vi "自动.vi"() -> ()   [LabVIEW 2017]
uses:
  <vilib>/Platform/TimedLoop/XDataNode/XDataNode.xnode
  <vilib>/Platform/TimedLoop/XDataNode/nitl_modes.ctl
  <vilib>/Platform/TimedLoop/XDataNode/XDNodeRunTimeDep.lvlib
  <vilib>/Platform/TimedLoop/XDataNode/wakeup.ctl
  <vilib>/Platform/TimedLoop/XDataNode/timing_clust.ctl
  <vilib>/rvi/interface/nirviCloseFPGA/nirviCloseFPGA.xnode
  <vilib>/myRIO/Instrument Drivers/Utilities/Utilities.lvlib
  <vilib>/FPGAPlugInAG/Dynamic/niLvFpga_Close_Dynamic.vi
panel:
  in  "开始":bool
  in  "枚举":enum16{"等待", "前进", "减速", "停止"}(ring)
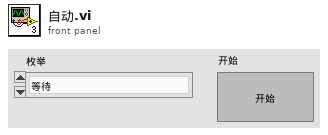
[diagram p1: front panel]
types:
  T1 = typedef "PWM.lvlib/PWM Reference.ctl" = cluster{"myRIO Reference":T2, "PWM Channels Enum":T6, "PWM Configuration":T7}
  T2 = typedef "myRIO Generic Hardware Reference.ctl" = cluster{"myRIO Model":T3, "myRIO Hardware Reference":T4}
  T3 = typedef "Hardware Version Enum.ctl" = enum16{"Unknown", "myRIO-1900", "myRIO-1950", "roboRIO", "NI ELVIS RIO CM"}
  T4 = typedef "myRIO v1.0 Reference.ctl" = cluster{"Generic FPGA Reference":T5, "Allow multiple opens":bool}
  T5 = typedef "Generic FPGA Reference.ctl" = refnum<k20>
  T6 = typedef "PWM Channels Enum.ctl" = enum16{"Not Connected", "C/PWM0", "C/PWM1", "A/PWM0", "A/PWM1", "A/PWM2", "B/PWM0", "B/PWM1", "B/PWM2", "PWM/PWM0", "PWM/PWM1", "PWM/PWM2", "PWM/PWM3", "PWM/PWM4", "PWM/PWM5", "PWM/PWM6", "PWM/PWM7", "PWM/PWM8", "PWM/PWM9"}
  T7 = typedef "PWM.lvlib/PWM Configuration.ctl" = cluster{"Frequency":dbl, "Duty Cycle":dbl}
  T8 = typedef "Encoder.lvlib/Encoder Reference.ctl" = cluster{"myRIO Reference":T2, "Encoder Channels Enum":T9}
  T9 = typedef "Encoder Channels Enum.ctl" = enum16{"Not Connected", "C/ENC0", "C/ENC1", "A/ENC", "B/ENC", "DIO/ENC0", "DIO/ENC1", "DIO/ENC2", "DIO/ENC3", "DIO/ENC4"}
  T10 = typedef "DIO.lvlib/DIO Reference.ctl" = cluster{"myRIO Reference":T2, "DIO Channels List":T11}
  T11 = typedef "DIO Channels List.ctl" = T12[]
  T12 = typedef "DIO Channels Enum.ctl" = enum16{"Not Connected", "C/DIO0", "C/DIO1", "C/DIO2", "C/DIO3", "C/DIO4", "C/DIO5", "C/DIO6", "C/DIO7", "A/DIO0", "A/DIO1", "A/DIO2", "A/DIO3", "A/DIO4", "A/DIO5", "A/DIO6", "A/DIO7", "A/DIO8", "A/DIO9", "A/DIO10", "A/DIO11", "A/DIO12", "A/DIO13", "A/DIO14", "A/DIO15", "B/DIO0", "B/DIO1", "B/DIO2", "B/DIO3", "B/DIO4", "B/DIO5", "B/DIO6", "B/DIO7", "B/DIO8", "B/DIO9", "B/DIO10", "B/DIO11", "B/DIO12", "B/DIO13", "B/DIO14", "B/DIO15", "LED0", "LED1", "LED2", "LED3", "Button0", "DIO/DIO0", "DIO/DIO1", "DIO/DIO2", "DIO/DIO3", "DIO/DIO4", "DIO/DIO5", "DIO/DIO6", "DIO/DIO7", "DIO/DIO8", "DIO/DIO9", "SPI/CS0", "SPI/CS1", "SPI/CS2", "SPI/CS3", "LED RADIO (Green)", "LED RADIO (Red)", "LED COMM (Green)", "LED COMM (Red)", "LED MODE (Green)", "LED MODE (Red)"}
  T13 = cluster{"PWM":T1[], "ENC":T8[], "DIO":T10, "FPGA Reference":refnum<k20>}
  T14 = typedef "XDNodeRunTimeDep.lvlib/timing_clust.ctl" = cluster{"Expected End [f-1]":u64, "Actual End [f-1]":u64, "Finished Late? [f-1]":bool, "Expected End [i-1]":u64, "Actual End [i-1]":u64, "Finished Late? [i-1]":bool, "Expected Start [i]":u64, "Actual Start [i]":u64, "Expected Start [f]":u64, "Actual Start [f]":u64, "Source Name":string, "Structure Name":string, "Period":i64, "Deadline":i64, "Offset":i64, "Start":i64, "Priority":i32, "Timeout":i32, "Mode":T15, "Wakeup Reason":T16, "Error":errorcluster, "Source Type":string, "Secondary Source Type":string, "Global End Time":u64, "Global Start Time":u64, "Frame Duration":u64, "Iteration Duration":u64, "Assigned CPU":i32, "I/O Scan Engine Mode":u32}
  T15 = typedef "XDNodeRunTimeDep.lvlib/nitl_modes.ctl" = enum32{"No Change", "Process missed periods, maintain original phase", "Discard missed periods, maintain original phase", "Process missed periods, ignore original phase", "Discard missed periods, ignore original phase"}
  T16 = typedef "XDNodeRunTimeDep.lvlib/wakeup.ctl" = enum32{"Normal", "Aborted", "Asynchronous wakeup", "Timing source error", "Timed loop error", "Timeout"}
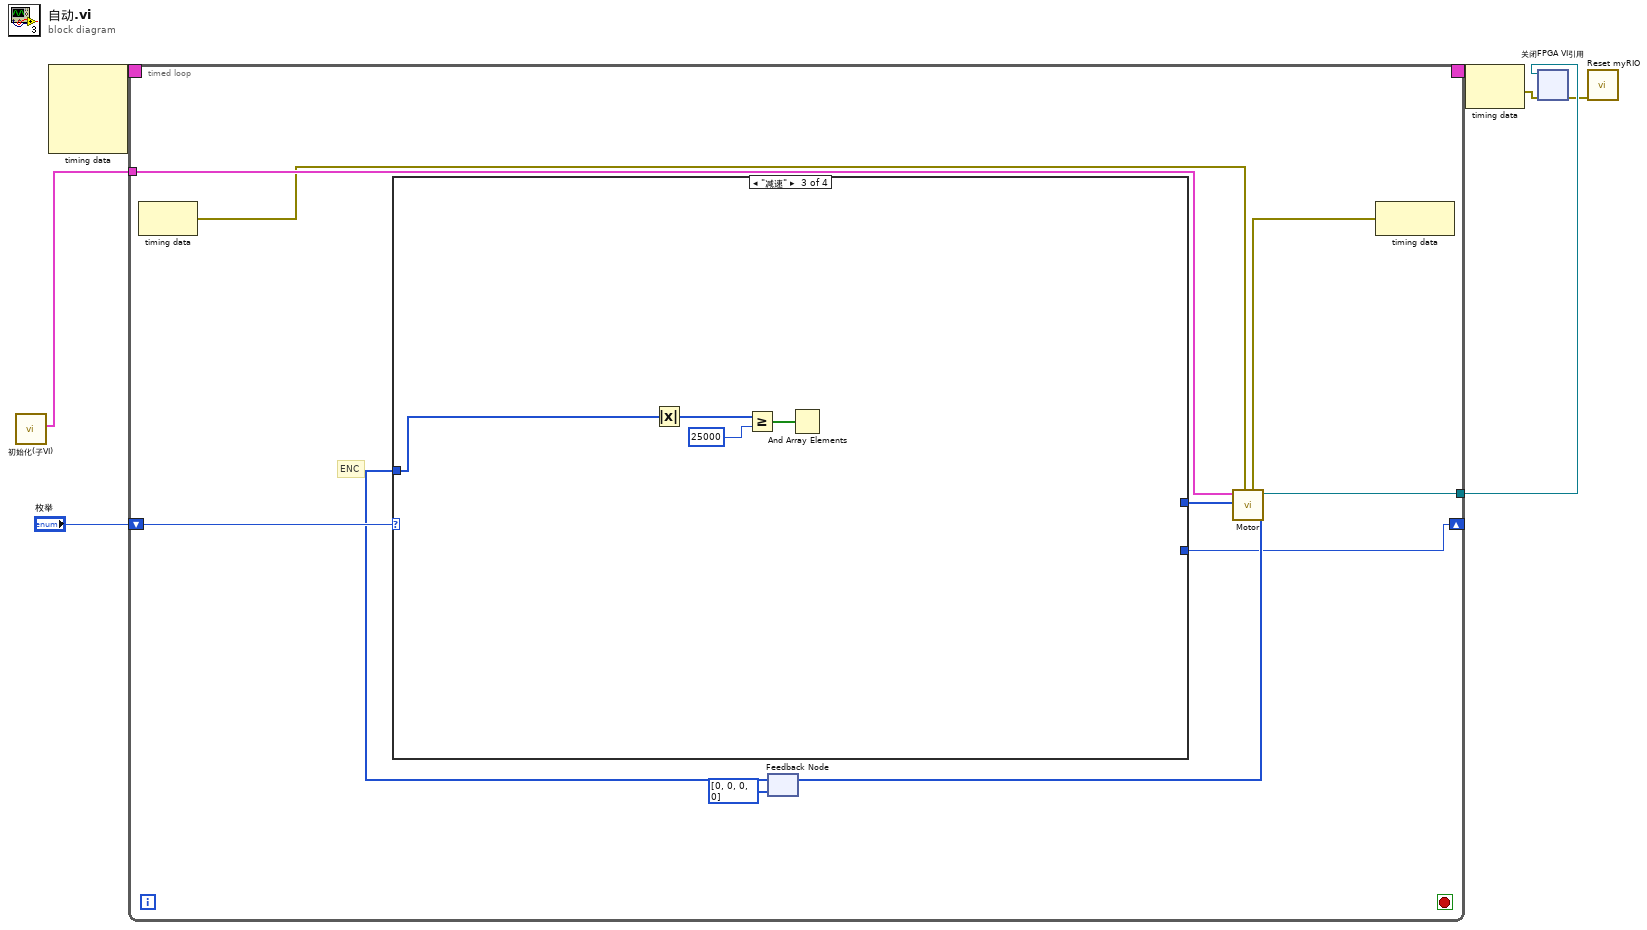
[diagram p0: block diagram]
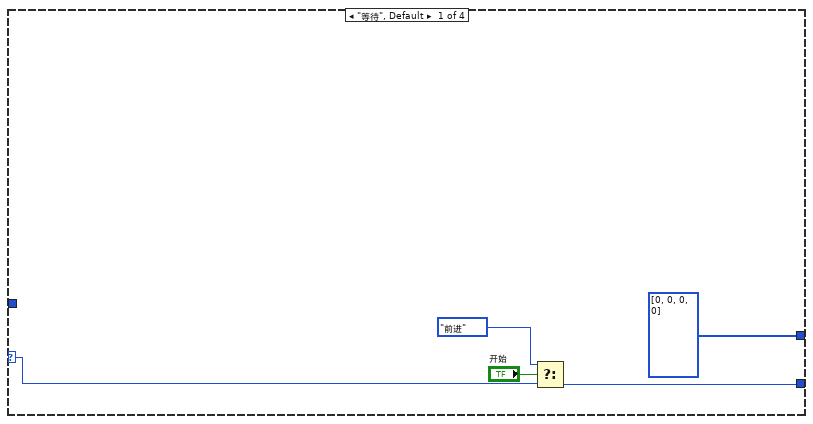
[diagram p2: hidden frame]
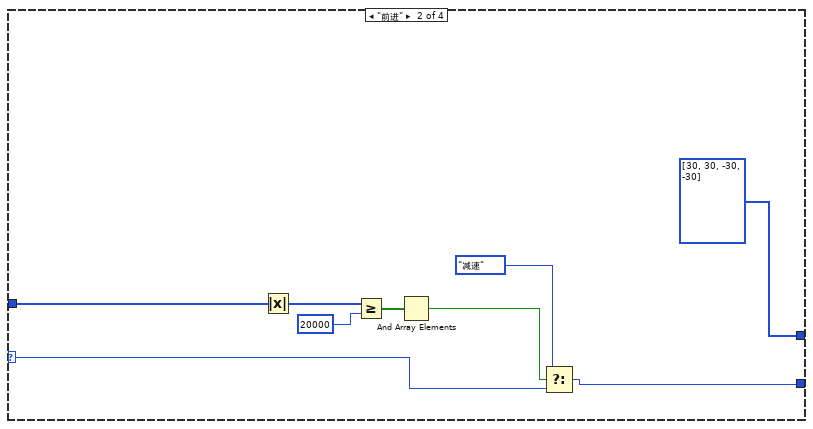
[diagram p3: hidden frame]
diagram:
  n1 = call "初始化(子VI).vi"() -> ("Reference"=w5:T13)  [unwired: 10 in, 1 out]
  n2 = node-c288() -> (w7:T14)  [unwired: 4 in]
  n3 = timed-loop {
    timing: w7 -> [_]
    timing-out: [_] -> w6
    tunnel: w5 -> [w17]
    tunnel: [w14] -> w3
    shift-right: [w8] -> _
    shift-left: "枚举" -> [w13]
    stop <- _ stop-if-true
    # "ENC"
    n4 = node-c288() -> (w16:errorcluster)  [unwired: 1 in]
    n5 = feedback #1(i32[] [0, 0, 0, 0] ("ENC")) -> (w10:i32[])
    n6 = case shown="\"减速\"" w13 {
      selector: w13 -> [w21 w25 _ _]
      tunnel: w10 -> [_ w30 w32 _]
      tunnel: [i32[] [0, 0, 0, 0] ("SET") i32[] [30, 30, -30, -30] ("SET") _ _] -> w11
      tunnel: [w20 w24 _ _] -> w8
      frame "等待", Default {
        n7 = Select(t=enum16{"等待", "前进", "减速", "停止"}."前进" ("枚举 2"), s="开始", f=w21) -> (s? t:f=w20:enum16{"等待", "前进", "减速", "停止"})
      }
      frame "前进" {
        n8 = Absolute Value(x=w30) -> (abs(x)=w28:i32[])
        n9 = Greater Or Equal?(x=w28, y=20000) -> (x >= y?=w27:bool[])
        n10 = And Array Elements(Boolean array=w27) -> (logical AND=w26:bool)
        n11 = Select(t=enum16{"等待", "前进", "减速", "停止"}."减速" ("枚举 2"), s=w26, f=w25) -> (s? t:f=w24:enum16{"等待", "前进", "减速", "停止"})
      }
      frame "减速" {
        n12 = Absolute Value(x=w32) -> (abs(x)=w34:i32[])
        n13 = Greater Or Equal?(x=w34, y=25000) -> (x >= y?=w33:bool[])
        n14 = And Array Elements(Boolean array=w33) -> ()  [unwired: 1 out]
      }
      frame "停止" {
      }
    }
    n15 = call "Motor.vi"("ERRI"=w16, "SET"=w11, "Reference"=w17) -> ("ENC"=w12:i32[], "FPGA VI引用输出"=w14:refnum<k20>, "ERRO"=w15:errorcluster)  [unwired: 6 in]
    n16 = feedback-in #1(w12) -> ()
    n17 = node-c288(w15) -> ()  [unwired: 1 out]
  }
  n18 = node-c288(w6) -> (w4:errorcluster)
  n19 = xnode "关闭FPGA VI引用"("FPGA VI引用输入"=w3, "错误输入"=w4) -> ("错误输出"=w2:errorcluster)
  n20 = call <vilib>:"Reset myRIO.vi"("error in (no error)"=w2) -> ()  [unwired: 10 in, 1 out]
